vi "Set message.vi"(10 "WampMessage JSON":refnum<class "WampMessage JSON.lvclass">, 11 "IJsonMessageHandler in":refnum<class "IJsonMessageHandler.lvclass">) -> (3 "IJsonMessageHandler out":refnum<class "IJsonMessageHandler.lvclass">)   [LabVIEW 2020, in "wamplv.lvlib" / "IJsonMessageHandler.lvclass"]
uses:
  IJsonMessageHandler.lvclass
  SerialisedMessages/JSONMessage/WampMessage JSON.lvclass
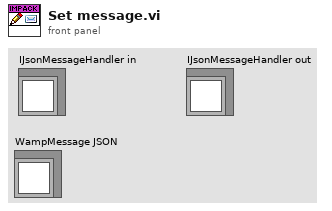
[diagram p1: front panel]
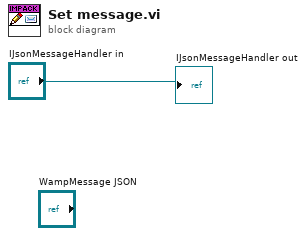
[diagram p0: block diagram]
diagram:
  "IJsonMessageHandler out" <- "IJsonMessageHandler in"
